vi "Range Maximum Write.vi"(6 "Control Ref Queue":T1, 8 "error in (no error)":errorcluster, 9 "Range Max":sgl, 11 "3D Plot.lvclass in":refnum<class "3D Plot.lvclass">) -> (0 "error out":errorcluster, 3 "3D Plot.lvclass out":refnum<class "3D Plot.lvclass">)   [LabVIEW 2020, in "3D Plot.lvclass"]
uses:
  3D Plot.lvclass
  3DMathPlot Ctrl Act Queue.ctl
  3DMathPlot Ctrl Act Cluster.ctl
  3DMathPlot State Class.ctl
  3D Plot.lvclass/3D Plot.ctl
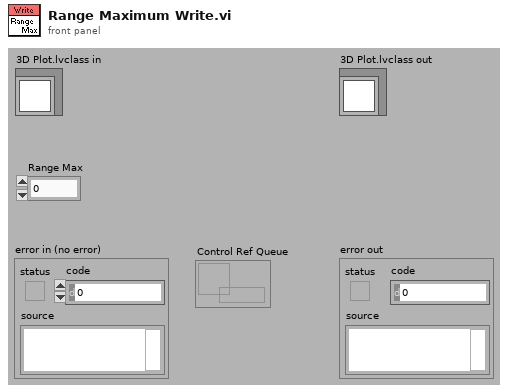
[diagram p1: front panel]
types:
  T1 = typedef "3DMathPlot Ctrl Act Queue.ctl" = refnum<queue>
  T2 = typedef "3D Plot.lvclass/Range Clusters.ctl" = cluster{"X Range":cluster{"Max X":sgl, "Min X":sgl}, "Y Range":cluster{"Max Y":sgl, "Min Y":sgl}, "Z Range":cluster{"Max Z":sgl, "Min Z":sgl}}
  T3 = cluster{"Auto Range X":bool, "Auto Range Y":bool, "Auto Range Z":bool}
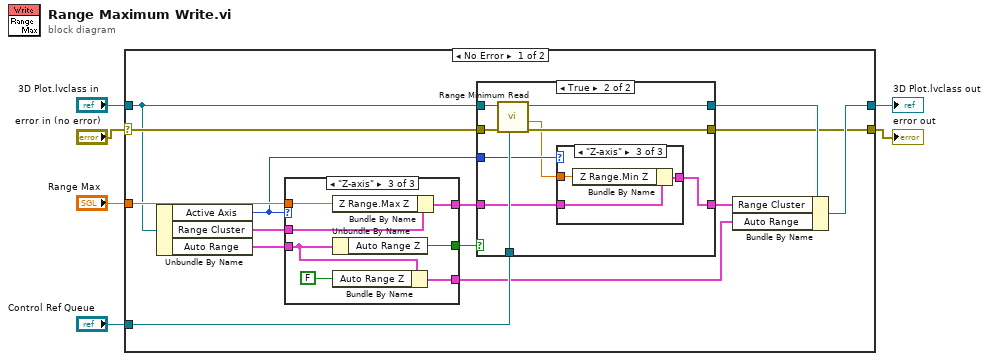
[diagram p0: block diagram]
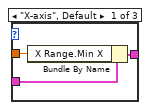
[diagram p3: hidden frame]
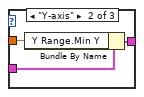
[diagram p4: hidden frame]
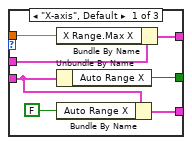
[diagram p5: hidden frame]
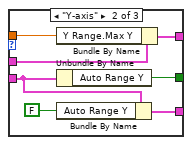
[diagram p6: hidden frame]
diagram:
  n1 = case shown="No Error" "error in (no error)" {
    selector: "error in (no error)" -> [w17 w63]
    tunnel: "Range Max" -> [w20 _]
    tunnel: "3D Plot.lvclass in" -> [w16 w64]
    tunnel: [w19 w64] -> w4
    tunnel: [w14 w63] -> w2
    tunnel: "Control Ref Queue" -> [w13 _]
    frame No Error {
      n2 = Unbundle By Name(w16) -> ("Active Axis"=w12:enum16{"X-axis", "Y-axis", "Z-axis"}, "Range Cluster"=w18:T2, "Auto Range"=w8:T3)
      n3 = case shown="\"Z-axis\"" w12 {
        tunnel: w18 -> [w48 w53 w60]
        tunnel: w20 -> [w47 w55 w62]
        tunnel: [w46 w54 w61] -> w11
        tunnel: w8 -> [w44 w50 w57]
        tunnel: [w45 w52 w59] -> w9
        tunnel: [w42 w49 w56] -> w7
        frame "X-axis", Default {
          n4 = Bundle By Name(cluster=w48, "X Range.Max X"=w47) -> (w46:T2)
          n5 = Unbundle By Name(w44) -> ("Auto Range X"=w45:bool)
          n6 = Bundle By Name(cluster=w44, "Auto Range X"=FALSE) -> (w42:T3)
        }
        frame "Y-axis" {
          n7 = Bundle By Name(cluster=w53, "Y Range.Max Y"=w55) -> (w54:T2)
          n8 = Unbundle By Name(w50) -> ("Auto Range Y"=w52:bool)
          n9 = Bundle By Name(cluster=w50, "Auto Range Y"=FALSE ("Auto Range X")) -> (w49:T3)
        }
        frame "Z-axis" {
          n10 = Bundle By Name(cluster=w60, "Z Range.Max Z"=w62) -> (w61:T2)
          n11 = Unbundle By Name(w57) -> ("Auto Range Z"=w59:bool)
          n12 = Bundle By Name(cluster=w57, "Auto Range Z"=FALSE ("Auto Range X")) -> (w56:T3)
        }
      }
      n13 = case shown="True" w9 {
        tunnel: w16 -> [w23 w32]
        tunnel: [w23 w31] -> w15
        tunnel: w17 -> [w22 w30]
        tunnel: [w22 w29] -> w14
        tunnel: w13 -> [_ w28]
        tunnel: w12 -> [_ w27]
        tunnel: w11 -> [w21 w26]
        tunnel: [w21 w25] -> w10
        frame False {
        }
        frame True {
          n14 = call "Range Minimum Read.vi"("Control Ref Queue"=w28, "error in (no error)"=w30, "3D Plot.lvclass in"=w32) -> ("error out"=w29:errorcluster, "Range Min"=w24:sgl, "3D Plot.lvclass out"=w31:refnum<class "3D Plot.lvclass">)  [unwired: 6 out]
          n15 = case shown="\"Z-axis\"" w27 {
            tunnel: w26 -> [w35 w38 w41]
            tunnel: [w33 w37 w39] -> w25
            tunnel: w24 -> [w34 w36 w40]
            frame "X-axis", Default {
              n16 = Bundle By Name(cluster=w35, "X Range.Min X"=w34) -> (w33:T2)
            }
            frame "Y-axis" {
              n17 = Bundle By Name(cluster=w38, "Y Range.Min Y"=w36) -> (w37:T2)
            }
            frame "Z-axis" {
              n18 = Bundle By Name(cluster=w41, "Z Range.Min Z"=w40) -> (w39:T2)
            }
          }
        }
      }
      n19 = Bundle By Name(cluster=w15, "Range Cluster"=w10, "Auto Range"=w7) -> (w19:refnum<class "3D Plot.lvclass">)
    }
    frame Error {
    }
  }
  "error out" <- w2
  "3D Plot.lvclass out" <- w4
